vi "Open TCP Session.vi"(8 "error in (no error)":errorcluster, 9 "Timeout (10000)":i32=10000, 10 "Port (502)":u16=502, 11 "IP Address":string="localhost") -> (0 "error out":errorcluster, 3 "MB_TCP session":refnum<class "MB_Master_TCP.lvclass">)   [LabVIEW 2012, in "MB Master.lvlib" / "MB_Master_TCP.lvclass"]
doc: "Opens a new modbus session and establish the TCP connection. Note that the slave ID is set to the default of 0xFF. Slave ID can be changed later via the property node \"Slave ID\"."
uses:
  MB_Master_TCP.lvclass
  MB_ADU/MB_ADU.lvclass/MB_ADU.ctl
  MB_ADU_TCP/MB_ADU_TCP.lvclass/MB_ADU_TCP.ctl
  MB_Master_TCP.lvclass/MB_Master_TCP.ctl
  MB_ADU/Build ADU.vi
  MB_ADU_TCP/MB_ADU_TCP.lvclass
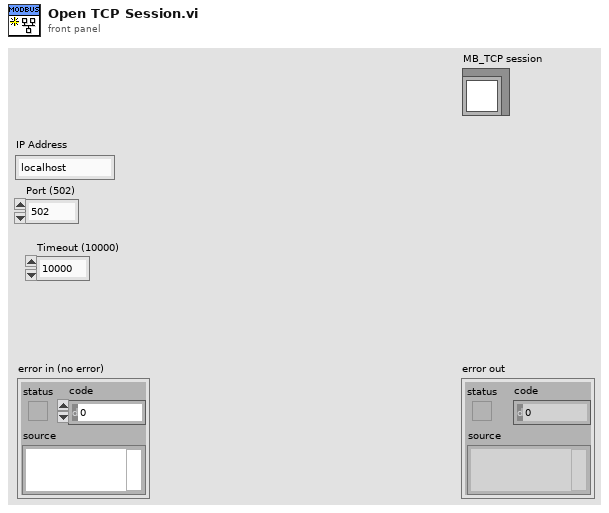
[diagram p1: front panel]
types:
  T1 = cluster{"IP Address":string, "Port":u16, "Timeout":i32, "Notifier":refnum<notifier>}
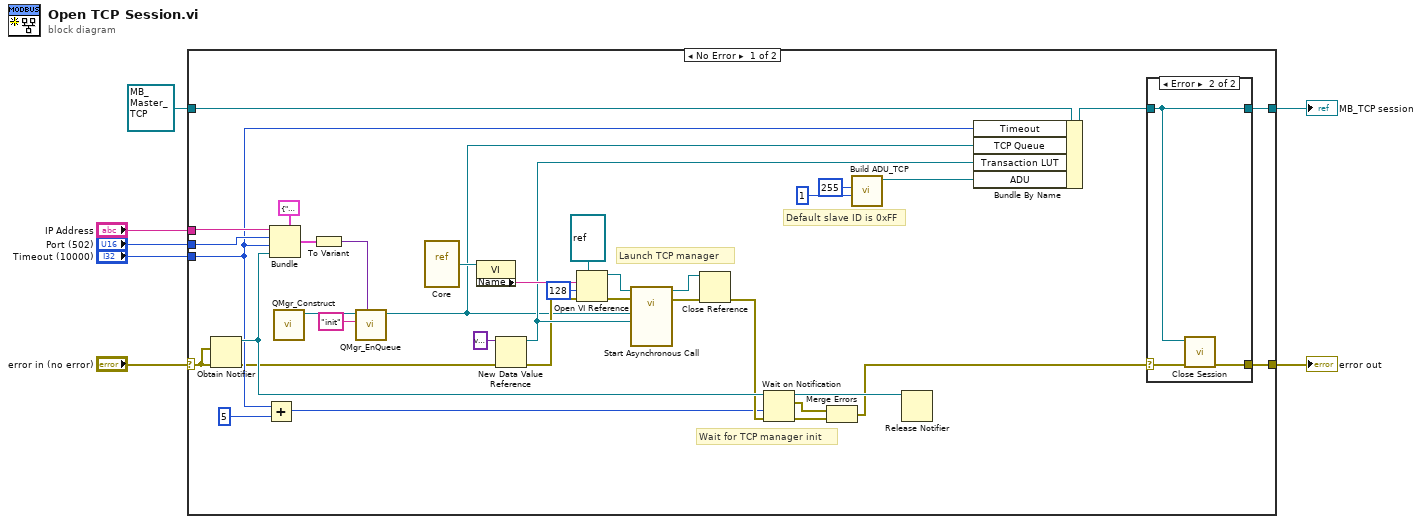
[diagram p0: block diagram]
diagram:
  n1 = case shown="No Error" "error in (no error)" {
    selector: "error in (no error)" -> [w20 w51]
    tunnel: [w24 w51] -> w6
    tunnel: [w26 w50] -> w4
    tunnel: refnum<class "MB_Master_TCP.lvclass"> refnum ("MB_Master_TCP in") -> [w44 w50]
    tunnel: "IP Address" -> [w39 _]
    tunnel: "Port (502)" -> [w38 _]
    tunnel: "Timeout (10000)" -> [w16 _]
    frame No Error {
      # "Wait for TCP manager init"
      # "Launch TCP manager"
      # "Default slave ID is 0xFF"
      n2 = Obtain Notifier(notification data type=w20, error in (no error)=w20) -> (notifier out=w29:refnum<notifier>, error out=w8:errorcluster)  [unwired: 2 in, 1 out]
      n3 = Add(x=w16, y=5) -> (x+y=w14:i32)
      n4 = Bundle(cluster=T1 {"IP Address"="", "Port"=502, "Timeout"=10000, "Notifier"=refnum}, "IP Address"=w39, "Port"=w38, "Timeout"=w16, "Notifier"=w29) -> (w31:T1)
      n5 = call "QMgr_Construct.vi"() -> ("queue out"=w12:refnum<queue>)  [unwired: 11 in]
      n6 = To Variant(anything=w31) -> (Variant=w10:variant)
      n7 = call "QMgr_EnQueue.vi"("Data"=w10, "Command"="init" ("cmd"), "queue in"=w12) -> ("queue out"=w9:refnum<queue>)  [unwired: 8 in]
      n8 = vi-ref "Core.vi"() -> (w33:refnum<vi>)
      n9 = property class="VI"(reference=w33) -> ("Name"=w34:string)  [unwired: 1 in, 2 out]
      n10 = New Data Value Reference(data value=variant ("variant"), error in=w8) -> (data value reference=w30:refnum<data-value>, error out=w19:errorcluster)
      n11 = Open VI Reference(type specifier VI Refnum (for type only)=refnum<vi> refnum, vi path=w34, options=128, error in (no error)=w19) -> (vi reference=w37:refnum<vi>, error out=w18:errorcluster)  [unwired: 2 in]
      n12 = call-by-ref "Start Asynchronous Call"(reference=w37, error in=w18, "Transaction LUT"=w30, "CMD Queue"=w9) -> (reference out=w23:refnum<vi>, error out=w22:errorcluster)  [unwired: 10 in]
      n13 = Close Reference(reference=w23, error in (no error)=w22) -> (error out=w21:errorcluster)
      n14 = Wait on Notification(notifier=w29, timeout in ms (-1)=w14, error in (no error)=w21) -> (notifier out=w17:refnum<notifier>, notification=w27:errorcluster, error out=w28:errorcluster)  [unwired: 1 in, 1 out]
      n15 = Merge Errors(w27, w28) -> (w13:errorcluster)
      n16 = call "Build ADU_TCP.vi"("Transaction ID"=u16 1, "Slave ID"=u8 255 ("Slave Address")) -> ("MB_ADU_TCP out"=w42:refnum<class "MB_ADU_TCP.lvclass">)  [unwired: 8 in, 1 out]
      n17 = Release Notifier(notifier=w17) -> ()  [unwired: 2 in, 3 out]
      n18 = Bundle By Name(cluster=w44, "Timeout"=w16, "TCP Queue"=w9, "Transaction LUT"=w30, "ADU"=w42) -> (w25:refnum<class "MB_Master_TCP.lvclass">)
      n19 = case shown="Error" w13 {
        selector: w13 -> [w45 w47]
        tunnel: [w46 w48] -> w26
        tunnel: w25 -> [w46 w48]
        tunnel: [w45 w49] -> w24
        frame No Error {
        }
        frame Error {
          n20 = call-dynamic "Close Session.vi"("error in (no error)"=w47, "MB TCP session"=w48) -> ("error out"=w49:errorcluster)  [unwired: 9 in]
        }
      }
    }
    frame Error {
    }
  }
  "error out" <- w6
  "MB_TCP session" <- w4
